vi "DrawMap.vi"(8 "error in (no error)":errorcluster, 10 "Map":i8[][](array[numeric]), 11 "picture":picture) -> (0 "error out":errorcluster, 3 "new picture":picture)   [LabVIEW 2009, in "Host.lvlib" / "Draw.lvlib"]
uses:
  Draw.lvlib
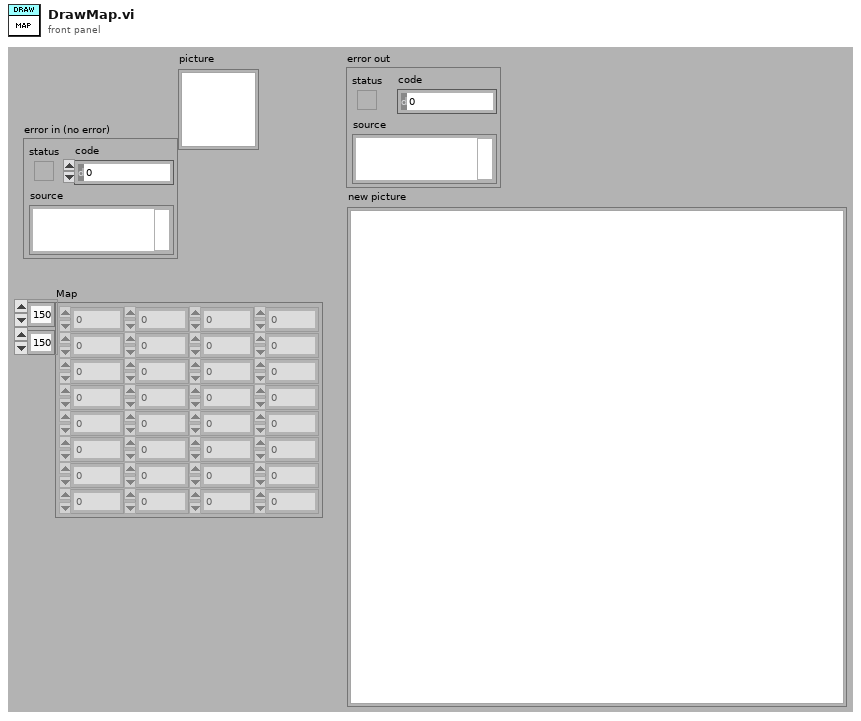
[diagram p1: front panel]
types:
  T1 = cluster{"Width":u16, "Style":enum32{"Solid", "Dash", "Dot", "DashDot", "DashDotDot"}}
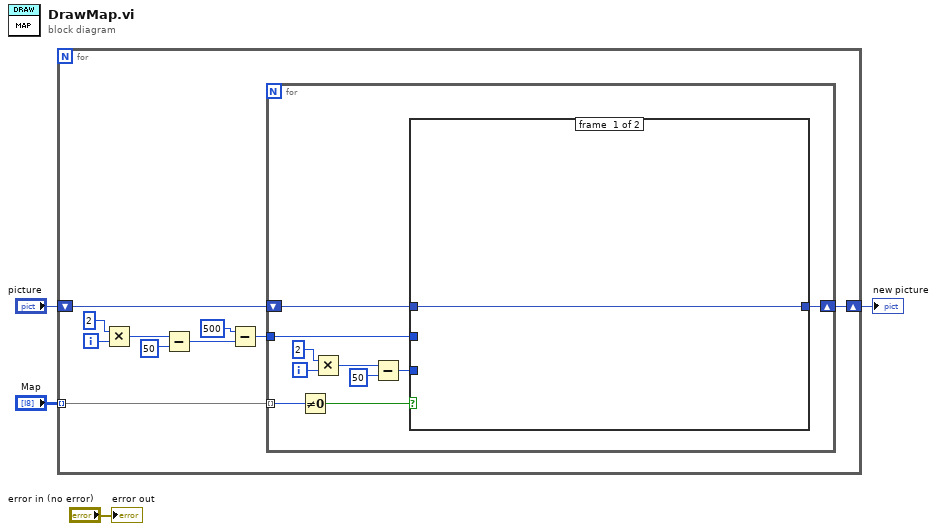
[diagram p0: block diagram]
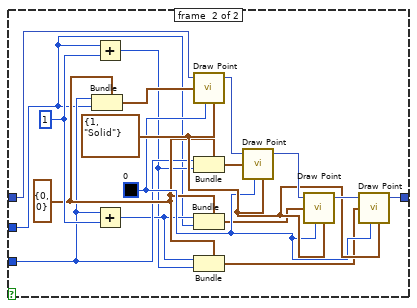
[diagram p2: hidden frame]
diagram:
  n1 = for {
    tunnel: "Map" -> [w14] mode=indexing
    shift-right: [w12] -> w1
    shift-left: "picture" -> [w13]
    i -> [w11]
    n2 = Multiply(x=2, y=w11) -> (x*y=w9:i32)
    n3 = Subtract(x=w9, y=50) -> (x-y=w7:i32)
    n4 = Subtract(x=500, y=w7) -> (x-y=w5:i32)
    n5 = for {
      tunnel: w14 -> [w23] mode=indexing
      tunnel: w5 -> [w22]
      shift-right: [w20] -> w12
      shift-left: w13 -> [w21]
      i -> [w19]
      n6 = Not Equal To 0?(x=w23) -> (x != 0?=w24:bool)
      n7 = Multiply(x=2, y=w19) -> (x*y=w17:i32)
      n8 = Subtract(x=w17, y=50) -> (x-y=w15:i32)
      n9 = case shown="True" w24 {
        tunnel: w22 -> [_ w26]
        tunnel: w15 -> [_ w29]
        tunnel: w21 -> [w25 w41]
        tunnel: [w25 w37] -> w20
        frame #0 {
        }
        frame #1 {
          w38 = 1 ("y")
          w34 = T1 {"Width"=1, "Style"=enum."Solid"} ("pen")
          w33 = u32 0 ("color(black)")
          w32 = cluster{"x":i16, "y":i16} {"x"=0, "y"=0} ("point(x,y)")
          n10 = Bundle(cluster=w32, "x"=w29, "y"=w26) -> (w42:cluster{"x":i16, "y":i16})
          n11 = Add(x=w26, y=w38) -> (x+y=w27:i32)
          n12 = Add(x=w29, y=w38) -> (x+y=w28:i32)
          n13 = call <vilib>:"Draw Point.vi"("picture"=w41, "point(x,y)"=w42, "color(black)"=w33, "pen"=w34) -> ("new picture"=w40:picture)  [unwired: 5 in]
          n14 = Bundle(cluster=w32, "x"=w29, "y"=w27) -> (w39:cluster{"x":i16, "y":i16})
          n15 = Bundle(cluster=w32, "x"=w28, "y"=w26) -> (w31:cluster{"x":i16, "y":i16})
          n16 = Bundle(cluster=w32, "x"=w28, "y"=w27) -> (w30:cluster{"x":i16, "y":i16})
          n17 = call <vilib>:"Draw Point.vi"("picture"=w40, "point(x,y)"=w39, "color(black)"=w33, "pen"=w34) -> ("new picture"=w35:picture)  [unwired: 5 in]
          n18 = call <vilib>:"Draw Point.vi"("picture"=w35, "point(x,y)"=w31, "color(black)"=w33, "pen"=w34) -> ("new picture"=w36:picture)  [unwired: 5 in]
          n19 = call <vilib>:"Draw Point.vi"("picture"=w36, "point(x,y)"=w30, "color(black)"=w33, "pen"=w34) -> ("new picture"=w37:picture)  [unwired: 5 in]
        }
      }
    }
  }
  "new picture" <- w1
  "error out" <- "error in (no error)"
